vi "Write Elevator Call.vi"(8 "error in (no error)":errorcluster, 10 "Elevator Call":T1, 11 "Sim User Console Actor in":refnum<class "Sim User Console Actor.lvclass">) -> (0 "error out":errorcluster, 3 "Sim User Console Actor out":refnum<class "Sim User Console Actor.lvclass">)   [LabVIEW 2019, in "Simulated User Console Actor.lvlib" / "Sim User Console Actor.lvclass"]
uses:
  Sim User Console Actor.lvclass
  Elevator Call.ctl
panel:
  # "Fourth Floor"
  # "Third Floor"
  # "Second Floor"
  # "First Floor"
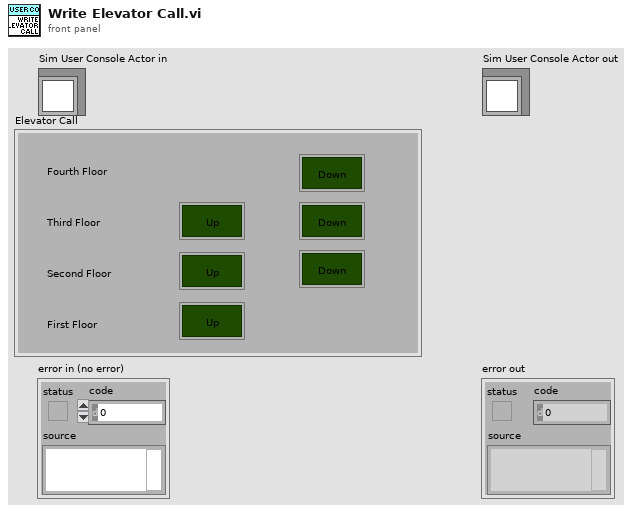
[diagram p1: front panel]
types:
  T1 = typedef "Simulated User Console Actor.lvlib/Sim User Console Actor.lvclass/Elevator Call.ctl" = cluster{"Up":bool, "Up 2":bool, "Up 3":bool, "Down":bool, "Down 2":bool, "Down 3":bool}
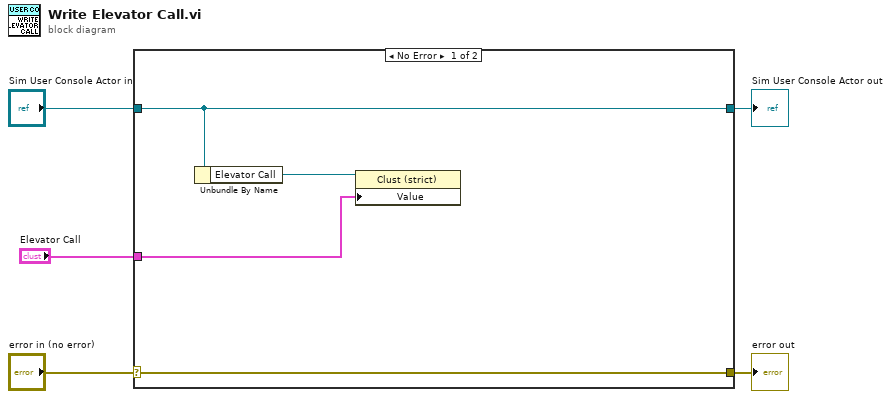
[diagram p0: block diagram]
diagram:
  n1 = case shown="No Error" "error in (no error)" {
    selector: "error in (no error)" -> [w9 w11]
    tunnel: [w9 w11] -> w4
    tunnel: [w8 w10] -> w2
    tunnel: "Sim User Console Actor in" -> [w8 w10]
    tunnel: "Elevator Call" -> [w6 _]
    frame No Error {
      n2 = Unbundle By Name(w8) -> ("Elevator Call"=w7:refnum<vi>)
      n3 = property class="Clust (strict)"(reference=w7, "Value"=w6) -> ()  [unwired: 1 in, 2 out]
    }
    frame Error {
    }
  }
  "error out" <- w4
  "Sim User Console Actor out" <- w2
